vi "Pins Disabled Read.vi"(4 "error in (no error)":errorcluster, 6 "Container State":T3, 7 "Display State In":T2) -> (0 "error out":errorcluster, 2 "Value":T1(array[ring]), 3 "Display State Out":T2)   [LabVIEW 2021, in "myRIO MXP.xctl"]
uses:
  <vilib>/myRIO/Common/Instrument Driver Framework/Utilities/xctls/myRIO MXP/myRIO MXP.xctl
  <vilib>/_xctls/Container State.ctl
  <vilib>/myRIO/Common/Instrument Driver Framework/Utilities/xctls/myRIO MXP/State.ctl
  <vilib>/_xctls/XControlSupport.lvlib
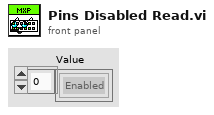
[diagram p1: front panel]
types:
  T1 = enum8{"Enabled", "Disabled", "Disabled and Grayed Out"}[]
  T2 = typedef "myRIO MXP.xctl/State.ctl" = cluster{"Pin Disabled?":enum8{"Enabled", "Disabled", "Disabled and Grayed Out"}[], "Pin Name":string[]}
  T3 = typedef "XControlSupport.lvlib/Container State.ctl" = cluster{"Indicator?":bool, "Run Mode?":bool, " Refnum":refnum<vi>}
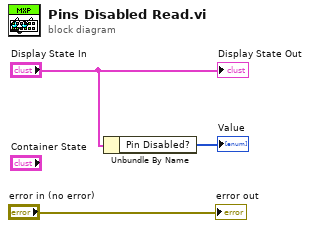
[diagram p0: block diagram]
diagram:
  n1 = Unbundle By Name("Display State In") -> ("Pin Disabled?"=→"Value":T1)
  "error out" <- "error in (no error)"
  "Display State Out" <- "Display State In"
